vi "Int SHVs.vi"(8 "error in (no error)":errorcluster, 11 "cRIO-CO2 in":refnum<class "cRIO-CO2.lvclass">) -> (0 "error out":errorcluster, 3 "cRIO-CO2 out":refnum<class "cRIO-CO2.lvclass">)   [LabVIEW 2015, in "cRIO-Carbondioxide.lvlib" / "cRIO-CO2.lvlib" / "cRIO-CO2.lvclass"]
uses:
  cRIO-CO2.lvclass
  Controls/Sample Transfer State Enumerator.ctl
  Controls/Sample Transfer Container Enumerator.ctl
  Controls/Sample Transfer Control Enumerator.ctl
  Controls/Sample Push Control Enumerator.ctl
  cRIO-CO2.lvclass/cRIO-CO2.ctl
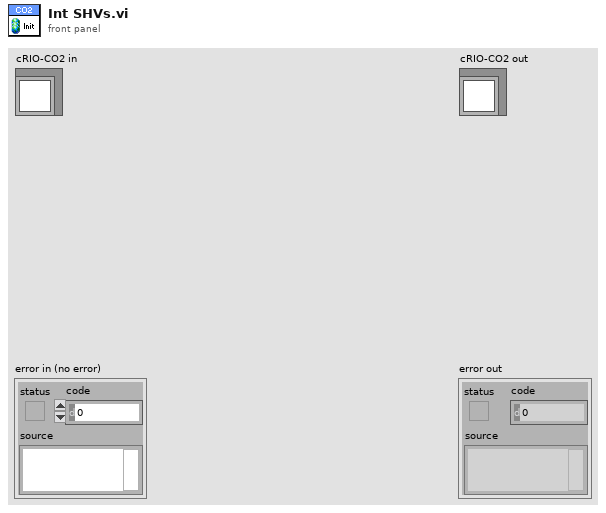
[diagram p1: front panel]
types:
  T1 = typedef "Sample Push Control Enumerator.ctl" = enum16{"Acknowledged", "Push", "Stash", "Abort", "Reset to Idle"}
  T2 = typedef "Sample Transfer Control Enumerator.ctl" = enum16{"Acknowledged", "Transfer", "Stash", "Abort", "Reset to Idle"}
  T3 = typedef "Sample Transfer Container Enumerator.ctl" = enum16{"None", "Sample 1", "Sample 2", "Sample 3", "Sample 4", "Sample 5", "Storage 01", "Storage 02", "Storage 03", "Storage 04", "Storage 05", "Storage 06", "Storage 07", "Storage 08", "Storage 09", "Storage 10", "Storage 11", "Storage 12", "Syringe", "Undefined"}
  T4 = typedef "Sample Transfer State Enumerator.ctl" = enum16{"Idle", "Initialize", "Check Containers", "Check Temperatures", "Start Turbo", "Warm Up Containers", "Prepare for purging", "Purge Capillary", "Purge", "Open Containers", "Introduce Sample", "Measure Base Pressure", "Home Syringe", "Start Freezer", "Freeze Target", "Crystalize", "Initiate Stash", "Stash", "Polish", "Stop Freezers", "Push Sample", "Complete", "Abort", "Error", "Undefined"}
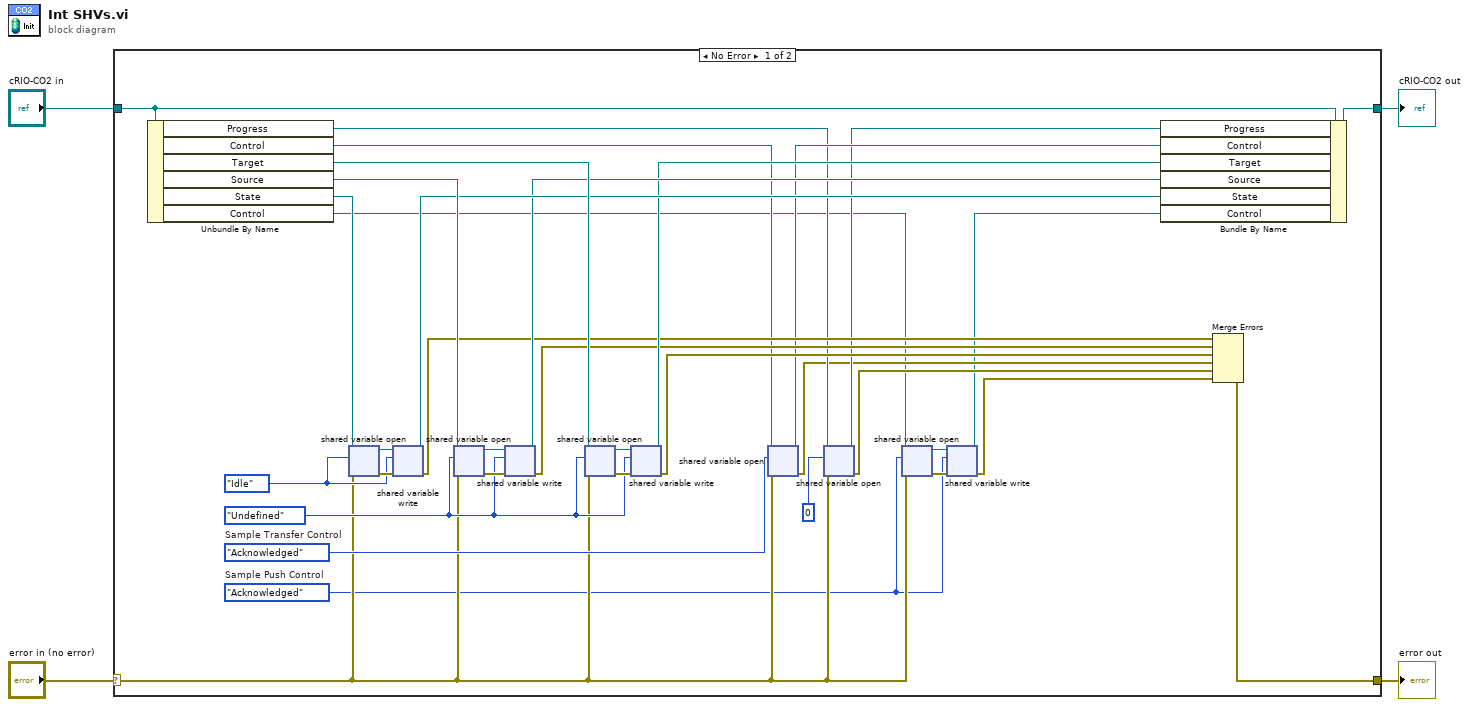
[diagram p0: block diagram]
diagram:
  n1 = case shown="No Error" "error in (no error)" {
    selector: "error in (no error)" -> [w11 w41]
    tunnel: [w21 w41] -> w3
    tunnel: [w38 w40] -> w1
    tunnel: "cRIO-CO2 in" -> [w20 w40]
    frame No Error {
      w9 = Sample_Push_Control_Enumerator."Acknowledged"  # Sample Push Control
      w18 = Sample_Transfer_Control_Enumerator."Acknowledged"  # Sample Transfer Control
      w27 = Sample_Transfer_Container_Enumerator."Undefined" ("Sample Transfer Container")
      w29 = Sample_Transfer_State_Enumerator."Idle" ("Sample Transfer State")
      n2 = Unbundle By Name(w20) -> ("Progress"=w16:refnum<k21>, "Control"=w19:refnum<k21>, "Target"=w36:refnum<k21>, "Source"=w37:refnum<k21>, "State"=w39:refnum<k21>, "Control"=w6:refnum<k21>)
      n3 = shared-variable-open(w39, w11, w29) -> (w34:refnum<k21>, w35:errorcluster)  [unwired: 1 in]
      n4 = shared-variable-write(w34, w35, w29) -> (w33:refnum<k21>, w24:errorcluster)
      n5 = shared-variable-open(w37, w11, w27) -> (w31:refnum<k21>, w32:errorcluster)  [unwired: 1 in]
      n6 = shared-variable-write(w31, w32, w27) -> (w30:refnum<k21>, w23:errorcluster)
      n7 = shared-variable-open(w36, w11, w27) -> (w26:refnum<k21>, w28:errorcluster)  [unwired: 1 in]
      n8 = shared-variable-write(w26, w28, w27) -> (w25:refnum<k21>, w22:errorcluster)
      n9 = shared-variable-open(w19, w11, w18) -> (w17:refnum<k21>, w13:errorcluster)  [unwired: 1 in]
      n10 = shared-variable-open(w16, w11, u8 0) -> (w15:refnum<k21>, w12:errorcluster)  [unwired: 1 in]
      n11 = shared-variable-open(w6, w11, w9) -> (w8:refnum<k21>, w10:errorcluster)  [unwired: 1 in]
      n12 = shared-variable-write(w8, w10, w9) -> (w5:refnum<k21>, w7:errorcluster)
      n13 = Bundle By Name(cluster=w20, "Progress"=w15, "Control"=w17, "Target"=w25, "Source"=w30, "State"=w33, "Control"=w5) -> (w38:refnum<class "cRIO-CO2.lvclass">)
      n14 = Merge Errors(w24, w23, w22, w13, w12, w7) -> (w21:errorcluster)
    }
    frame Error {
    }
  }
  "error out" <- w3
  "cRIO-CO2 out" <- w1
